vi "strip path example.vi"() -> ()   [LabVIEW 2016]
uses:
  <userlib>/_OpenG.lib/file/file.llb/Strip Path - Traditional__ogtk.vi
panel:
  out "name":string
  out "stripped path":path
  in  "path":path
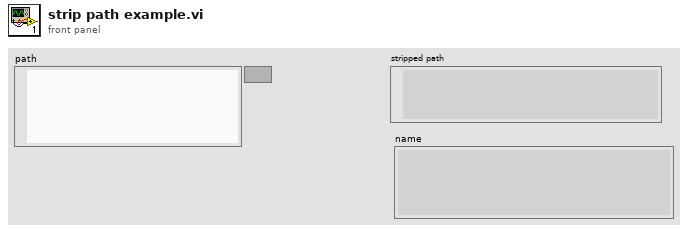
[diagram p1: front panel]
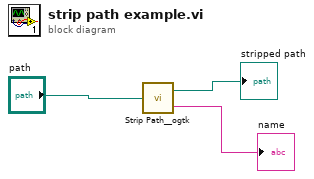
[diagram p0: block diagram]
diagram:
  n1 = call-poly <userlib>:"Strip Path__ogtk.vi"("path"="path") -> ("stripped path"=→"stripped path":path, "name"=→"name":string)
